vi "BigMAQ.vi"() -> ()   [LabVIEW 2019]
panel:
  in  "IDs":T1
  out "Names":string[](array[string])
  in  "Status State":string="UI: Status"
  in  "Status":string
  out "States Out 2":string
  out "States Out":string
  out "Current State 2":string
  out "Arguments":string
  out "Current State":string
  out "Numeric 2":dbl
  out "Numeric":dbl
  in  "Image Data Range":cluster{dbl, dbl}(slide)={100.0, 0.0} scale=0.0..100.0
  out "SVG Object":T2
  in  "Name":string
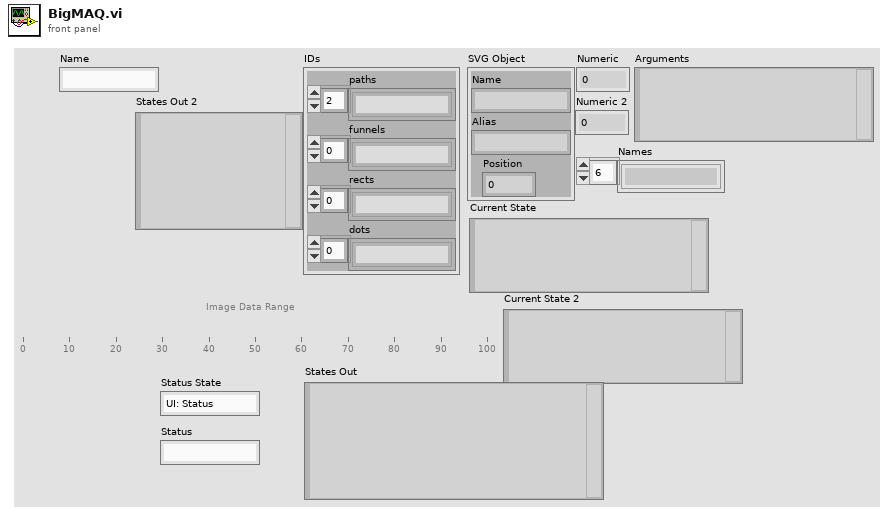
[diagram p1: front panel]
types:
  T1 = cluster{"paths":string[], "funnels":string[], "rects":string[], "dots":string[]}
  T2 = cluster{"Name":string, "Alias":string, "Position":i32}
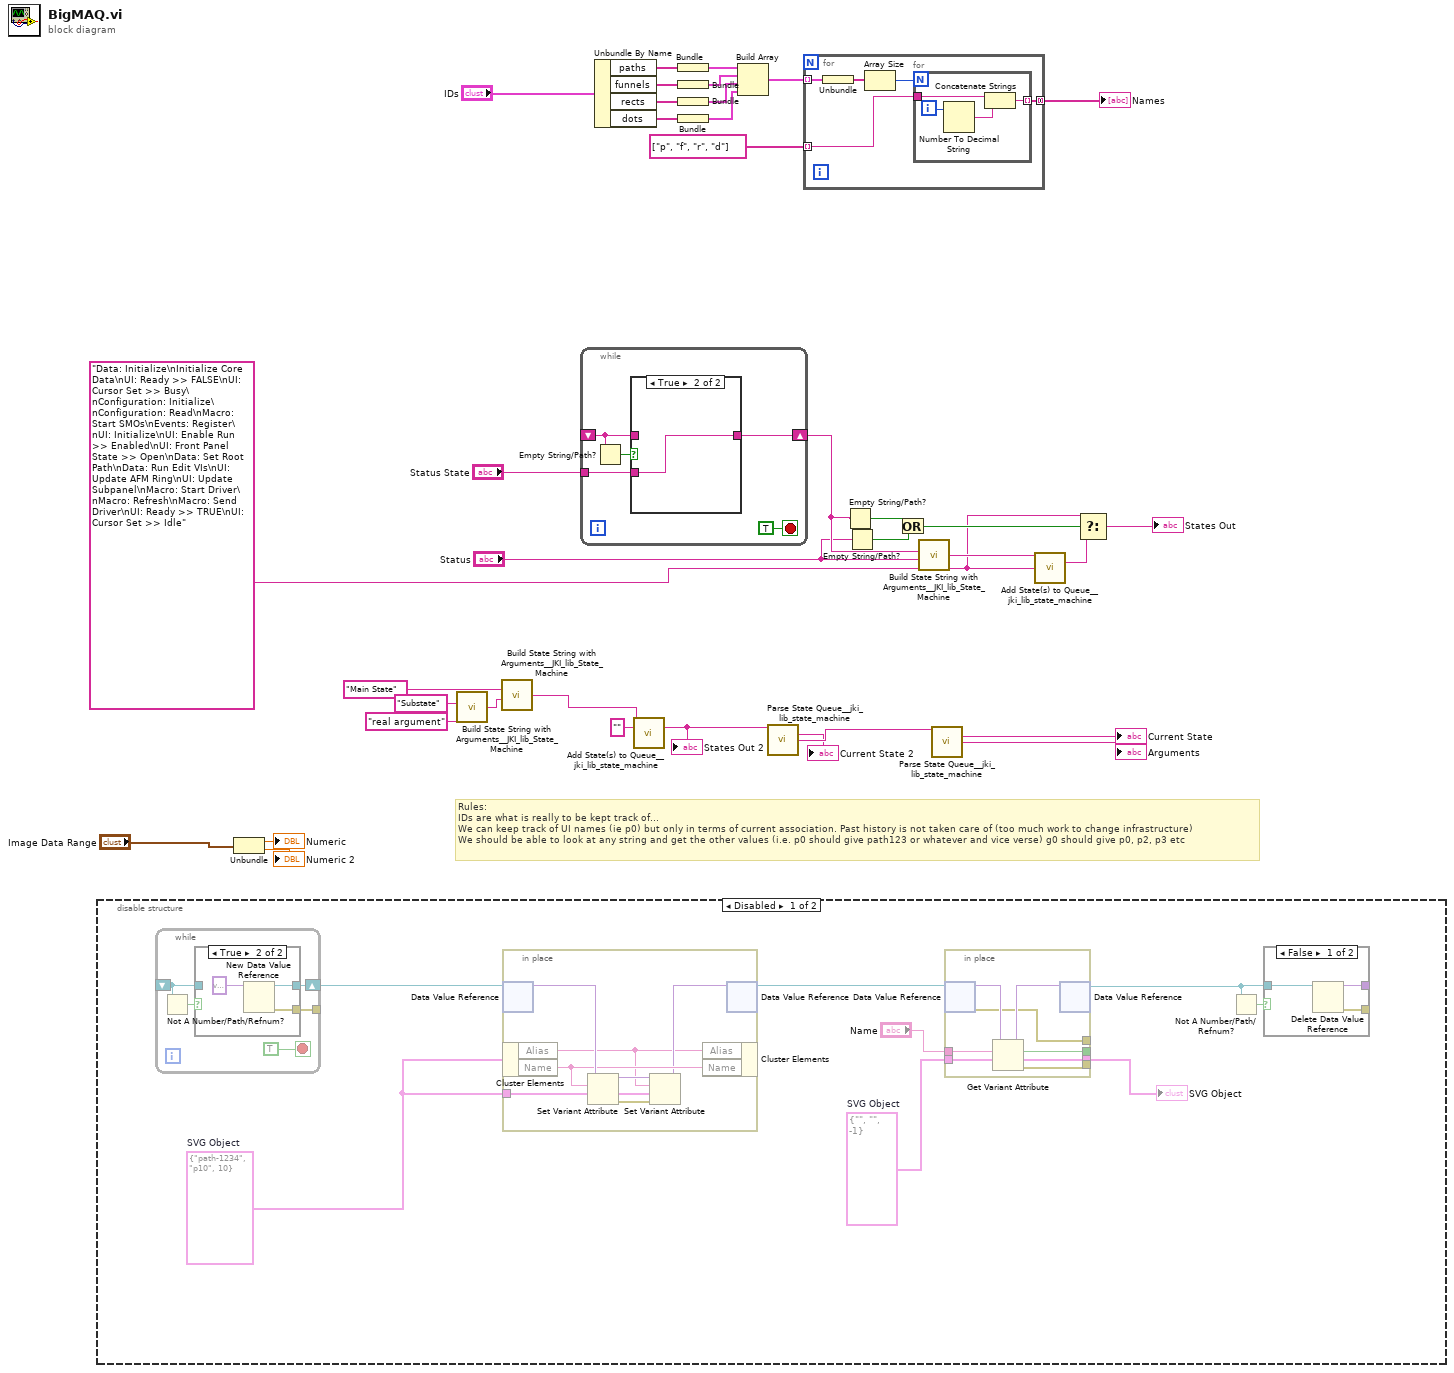
[diagram p0: block diagram]
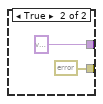
[diagram p3: hidden frame]
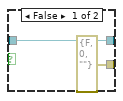
[diagram p4: hidden frame]
diagram:
  w13 = "Data: Initialize\nInitialize Core Data\nUI: Ready >> FALSE\nUI: Cursor Set >> Busy\nConfiguration: Initialize\nConfiguration: Read\nMacro: Start SMOs\nEvents: Register\nUI: Initialize\nUI: Enable Run >> Enabled\nUI: Front Panel State >> Open\nData: Set Root Path\nData: Run Edit VIs\nUI: Update AFM Ring\nUI: Update Subpanel\nMacro: Start Driver\nMacro: Refresh\nMacro: Send Driver\nUI: Ready >> TRUE\nUI: Cursor Set >> Idle"
  # "Rules:\nIDs are what is really to be kept track of... \nWe can keep track of UI names (ie p0) but only in terms of current association. Past history is not taken care of (too much work to change infrastructure)\nWe should be able to look at any string and get the other values (i.e. p0 should give path123 or whatever and vice verse) g0 should give p0, p2, p3 etc"
  n1 = disable-structure shown="Disabled" {
    frame Disabled {
      w37 = T2 {"Name"="path-1234", "Alias"="p10", "Position"=10}  # SVG Object
      w41 = T2 {"Name"="", "Alias"="", "Position"=-1}  # SVG Object
      n2 = while {
        shift-right: [w68] -> w40
        shift-left: _ -> [w66]
        tunnel: [w65] -> _
        stop <- TRUE stop-if-true
        n3 = Not A Number/Path/Refnum?(number/path/refnum=w66) -> (NaN/Path/Refnum?=w69:bool)
        n4 = case shown="True" w69 {
          tunnel: w66 -> [w71 _]
          tunnel: [w71 w73] -> w68
          tunnel: [errorcluster {"status"=FALSE, "code"=0, "source"=""} ("error out") w72] -> w65
          frame False {
          }
          frame True {
            n5 = New Data Value Reference(data value=variant) -> (data value reference=w73:refnum<data-value>, error out=w72:errorcluster)  [unwired: 1 in]
          }
        }
      }
      n6 = in-place {
        in-place-border: w37 -> [w45]
        n7 = in-place-dvr #1(w40) -> (w51:variant)  [unwired: 1 out]
        n8 = in-place-cluster #2(w37) -> ("Alias"=w46:string, "Name"=w50:string)
        n9 = Set Variant Attribute(Variant=w51, name=w50, value=w45) -> (Variant out=w48:variant, error out=w49:errorcluster)  [unwired: 1 in, 1 out]
        n10 = Set Variant Attribute(Variant=w48, name=w46, value=w45, error in=w49) -> (Variant out=w47:variant)  [unwired: 2 out]
        n11 = in-place-cluster #2("Alias"=w46, "Name"=w50) -> ()  [unwired: 1 out]
        n12 = in-place-dvr #1(w47) -> (w39:refnum<data-value>)  [unwired: 1 out]
      }
      n13 = in-place {
        in-place-border: [w64] -> w38
        in-place-border: "Name" -> [w61]
        in-place-border: w41 -> [w60]
        in-place-border: [w59] -> _
        in-place-border: [w58] -> _
        in-place-border: [w57] -> _
        n14 = in-place-dvr #3(w39) -> (w63:variant, w58:errorcluster)
        n15 = Get Variant Attribute(Variant=w63, name=w61, default value (empty Variant)=w60) -> (duplicate Variant=w62:variant, found=w59:bool, value=w64:T2, error out=w57:errorcluster)  [unwired: 1 in]
        n16 = in-place-dvr #3(w62) -> (w42:refnum<data-value>)  [unwired: 1 out]
      }
      "SVG Object" <- w38
      n17 = Not A Number/Path/Refnum?(number/path/refnum=w42) -> (NaN/Path/Refnum?=w43:bool)
      n18 = case shown="False" w43 {
        tunnel: w42 -> [w54 _]
        tunnel: [w52 errorcluster {"status"=FALSE, "code"=0, "source"=""} ("error out")] -> _
        tunnel: [w53 variant] -> _
        frame False {
          n19 = Delete Data Value Reference(data value reference=w54) -> (data value=w53:variant, error out=w52:errorcluster)  [unwired: 1 in]
        }
        frame True {
        }
      }
    }
    frame Enabled {
    }
  }
  n20 = Unbundle("Image Data Range") -> (→"Numeric":dbl, →"Numeric 2":dbl)
  n21 = call <vilib>:"Build State String with Arguments__JKI_lib_State_Machine.vi"("Arguments (\"\")"="real argument" ("Arguments (\"\")"), "State"="Substate") -> ("State with Arguments"=w29:string)  [unwired: 4 in]
  n22 = call <vilib>:"Build State String with Arguments__JKI_lib_State_Machine.vi"("Arguments (\"\")"=w29, "State"="Main State") -> ("State with Arguments"=w26:string)  [unwired: 4 in]
  n23 = while {
    tunnel: "Status State" -> [w77]
    shift-right: [w78] -> w20
    shift-left: _ -> [w75]
    stop <- TRUE stop-if-true
    n24 = Empty String/Path?(string/path=w75) -> (empty?=w76:bool)
    n25 = case shown="True" w76 {
      tunnel: [w80 w81] -> w78
      tunnel: w77 -> [_ w81]
      tunnel: w75 -> [w80 _]
      frame False {
      }
      frame True {
      }
    }
  }
  n26 = Unbundle By Name("IDs") -> ("paths"=w11:string[], "funnels"=w10:string[], "rects"=w9:string[], "dots"=w8:string[])
  n27 = call <vilib>:"Add State(s) to Queue__jki_lib_state_machine.vi"("State(s) in Front (\"\")"=w26, "State(s) in (\"\")"="" ("State(s) in (\"\")")) -> ("States Out"=w33:string)  [unwired: 13 in]
  "States Out 2" <- w33
  n28 = Bundle("paths"=w11) -> (w7:cluster{"paths":string[]})  [unwired: 1 in]
  n29 = Bundle("funnels"=w10) -> (w6:cluster{"funnels":string[]})  [unwired: 1 in]
  n30 = Bundle("rects"=w9) -> (w5:cluster{"rects":string[]})  [unwired: 1 in]
  n31 = Bundle("dots"=w8) -> (w4:cluster{"dots":string[]})  [unwired: 1 in]
  n32 = Build Array(w7, w6, w5, w4) -> (w2:cluster{"dots":string[]}[])
  n33 = call <vilib>:"Parse State Queue__jki_lib_state_machine.vi"("State Queue"=w33) -> ("Current State"=→"Current State 2":string, "Arguments"=w24:string)  [unwired: 12 in, 1 out]
  n34 = for {
    tunnel: string[] ["p", "f", "r", "d"] -> [w83] mode=indexing
    tunnel: w2 -> [w86] mode=indexing
    tunnel: [w82] -> w1 mode=concatenating
    n35 = Unbundle(w86) -> ("dots"=w85:string[])
    n36 = Array Size(array=w85) -> (size(s)=w84:i32)
    n37 = for {
      N: w84 -> [_]
      tunnel: w83 -> [w89]
      tunnel: [w87] -> w82 mode=indexing
      i -> [w90]
      n38 = Number To Decimal String(number=w90) -> (decimal integer string=w88:string)  [unwired: 1 in]
      n39 = Concatenate Strings(w89, w88) -> (w87:string)
    }
  }
  "Names" <- w1
  n40 = Empty String/Path?(string/path=w20) -> (empty?=w18:bool)
  n41 = Empty String/Path?(string/path="Status") -> (empty?=w17:bool)
  n42 = Or(x=w18, y=w17) -> (x .or. y?=w16:bool)
  n43 = call <vilib>:"Build State String with Arguments__JKI_lib_State_Machine.vi"("Arguments (\"\")"="Status", "State"=w20) -> ("State with Arguments"=w21:string)  [unwired: 4 in]
  n44 = call <vilib>:"Parse State Queue__jki_lib_state_machine.vi"("State Queue"=w24) -> ("Current State"=→"Current State":string, "Arguments"=→"Arguments":string)  [unwired: 12 in, 1 out]
  n45 = call <vilib>:"Add State(s) to Queue__jki_lib_state_machine.vi"("State(s) in Front (\"\")"=w21, "State(s) at Back (\"\")"=w13) -> ("States Out"=w15:string)  [unwired: 13 in]
  n46 = Select(t=w13, s=w16, f=w15) -> (s? t:f=→"States Out":string)
